vi "Encapsulation_Control.vi"(8 "error in":errorcluster, 11 "Encapsulation  State":bool) -> (0 "error out":errorcluster)   [LabVIEW 2016]
uses:
  <vilib>/DAQmx/write.llb/DAQmx Write (Digital Bool 1Line 1Point).vi
  <vilib>/DAQmx/create/channels.llb/DAQmx Create Channel (DO-Digital Output).vi
  <vilib>/DAQmx/miscellaneous.llb/DAQmx Fill In Error Info.vi
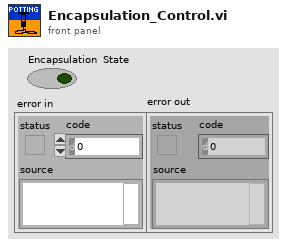
[diagram p1: front panel]
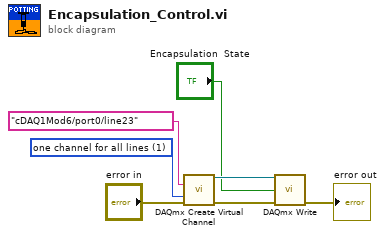
[diagram p0: block diagram]
diagram:
  w6 = 1 items=["one channel for each line", "one channel for all lines"] ("line grouping")
  n1 = call-poly <vilib>:"DAQmx Create Virtual Channel.vi"("lines"=tag "cDAQ1Mod6/port0/line23" ("Lines"), "line grouping"=w6, "error in"="error in") -> ("task out"=w5:refnum<k21>, "error out"=w4:errorcluster)  [unwired: 2 in, 9 out]
  n2 = call-poly <vilib>:"DAQmx Write.vi"("task/channels in"=w5, "data"="Encapsulation  State", "error in"=w4) -> ("error out"=→"error out":errorcluster)  [unwired: 1 in, 11 out]
